vi "workbook.create_free.vi"(8 "error in":errorcluster, 11 "WorkbookCreateStaging in":refnum<class "WorkbookCreateStaging.lvclass">) -> (0 "error out":errorcluster, 3 "WorkbookCreateStaging out":refnum<class "WorkbookCreateStaging.lvclass">)   [LabVIEW 2020, in "WorkbookCreateStaging.lvclass"]
doc: "Releases the handle and its associated resources."
uses:
  WorkbookCreateStaging.lvclass
  WorkbookCreateStaging.lvclass/WorkbookCreateStaging.ctl
  client.lvlib
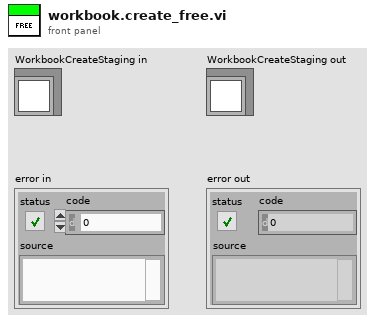
[diagram p1: front panel]
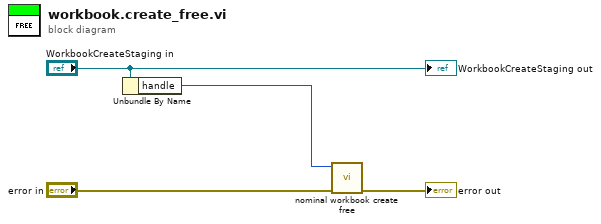
[diagram p0: block diagram]
diagram:
  n1 = Unbundle By Name("WorkbookCreateStaging in") -> ("handle"=w2:i32)
  n2 = call "nominal workbook create free.vi"("error in (no error)"="error in", "staging"=w2) -> ("error out"=→"error out":errorcluster)  [unwired: 8 in, 1 out]
  "WorkbookCreateStaging out" <- "WorkbookCreateStaging in"
